vi "obtain GFG_core VI Ref.vi"(11 "file path (use dialog)":path) -> (3 "GFG Refnum":refnum<vi>)   [LabVIEW 2012, in "GFG library.lvlib"]
doc: "SciScan 1.2 160622"
uses:
  GFG library.lvlib
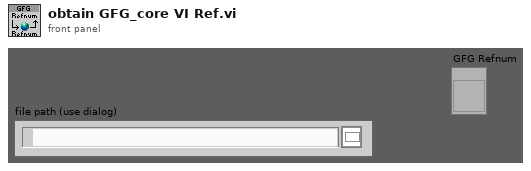
[diagram p1: front panel]
types:
  T1 = enum16{"open", "replace", "create", "open or create", "replace or create", "replace or create with confirmation"}
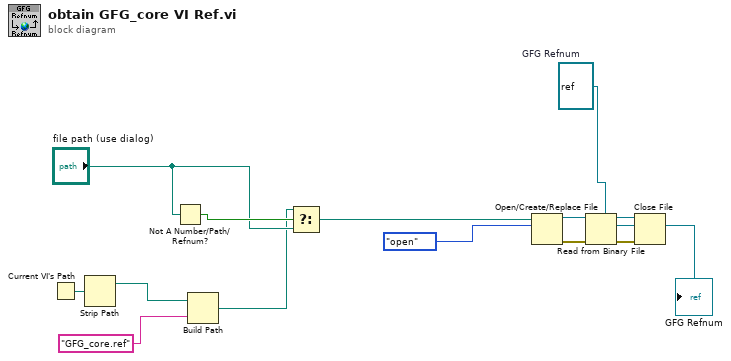
[diagram p0: block diagram]
diagram:
  w2 = refnum<vi> refnum  # GFG Refnum
  n1 = Current VI's Path() -> (path=w9:path)
  n2 = Strip Path(path=w9) -> (stripped path=w8:path)  [unwired: 1 out]
  n3 = Not A Number/Path/Refnum?(number/path/refnum="file path (use dialog)") -> (NaN/Path/Refnum?=w6:bool)
  n4 = Build Path(base path=w8, name or relative path="GFG_core.ref" ("replace string (\"\")")) -> (appended path=w4:path)
  n5 = Select(t=w4, s=w6, f="file path (use dialog)") -> (s? t:f=w3:path)
  n6 = Open/Create/Replace File(file path (use dialog)=w3, operation (0:open)=T1."open") -> (refnum out=w12:refnum<file>, error out=w13:errorcluster)  [unwired: 4 in, 1 out]
  n7 = Read from Binary File(5:w2, 8:w13, 11:w12) -> (0:w10:errorcluster, 2:→"GFG Refnum":refnum<vi>, 3:w11:refnum<file>)  [unwired: 3 in, 1 out]
  n8 = Close File(refnum=w11, error in=w10) -> ()  [unwired: 2 out]
